vi "HDF5_Init_ADAM_Refs.vi"(5 "HDF5 file ref":T2 format="%.0x", 9 "File Exists?":bool, 11 "error in":errorcluster) -> (4 "Health_Refs":T1 {"Group_ref" format="%.0x"; "ADAM_CoPol_dset" format="%.0x"; "ADAM_XPol_dset" format="%.0x"; "ADAM_Noise_dset" format="%.0x"; "ADAM_CalBox_dset" format="%.0x"; "TimeStamp" format="%.0x"}, 15 "error out":errorcluster)   [LabVIEW 2018]
doc: "Set up the HDF5 data structure and initialize the references for the Noise1, Noise2, Noise3, and Noise4 Datasets (tables).\n\nData structure:\nNoise1 (Dataset) - 1024 element Double array (waveform) \nNoise2 (Dataset) - 1024 element Double array (waveform) \nNoise3 (Dataset) - 1024 element Double array (waveform) \nNoise4 (Dataset) - 1024 element Double array (waveform)"
uses:
  <vilib>/addons/h5labview2/base/hid_t.ctl
  HDF5_ADAM_Refs.ctl
  HDF5_ADAM_Data.ctl
  lib_path_mod_20200519.vi
  <vilib>/addons/h5labview2/base/H5Equery.vi
  <vilib>/addons/h5labview2/attrib/H5Awrite.llb/H5Awrite.xnode
  <vilib>/addons/h5labview2/group/H5G.lvlib
  <vilib>/addons/h5labview2/dataset/H5D.lvlib
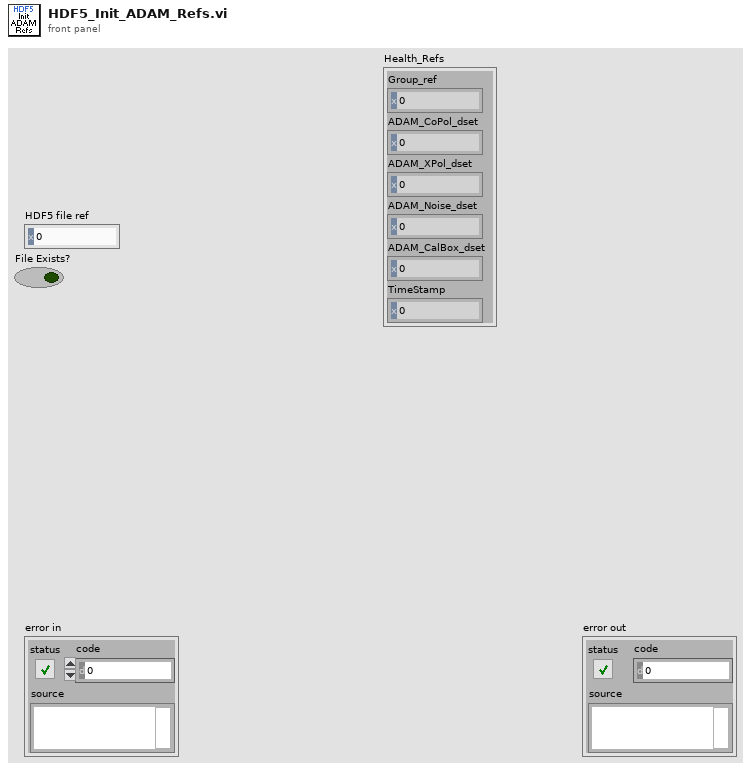
[diagram p1: front panel]
types:
  T1 = typedef "HDF5_ADAM_Refs.ctl" = cluster{"Group_ref":T2, "ADAM_CoPol_dset":T2, "ADAM_XPol_dset":T2, "ADAM_Noise_dset":T2, "ADAM_CalBox_dset":T2, "TimeStamp":T2}
  T2 = typedef "hid_t.ctl" = i32
  T3 = typedef "HDF5_ADAM_Data.ctl" = cluster{"Timestamp":dbl, "Time string":string, "Fault 1":bool, "Fault 2":bool, "Fault 3":bool, "Fault 4":bool, "Fault 5":bool, "Fault 6":bool, "Value 1":dbl, "Value 2":dbl, "Value 3":dbl, "Value 4":dbl, "Value 5":dbl, "Value 6":dbl}
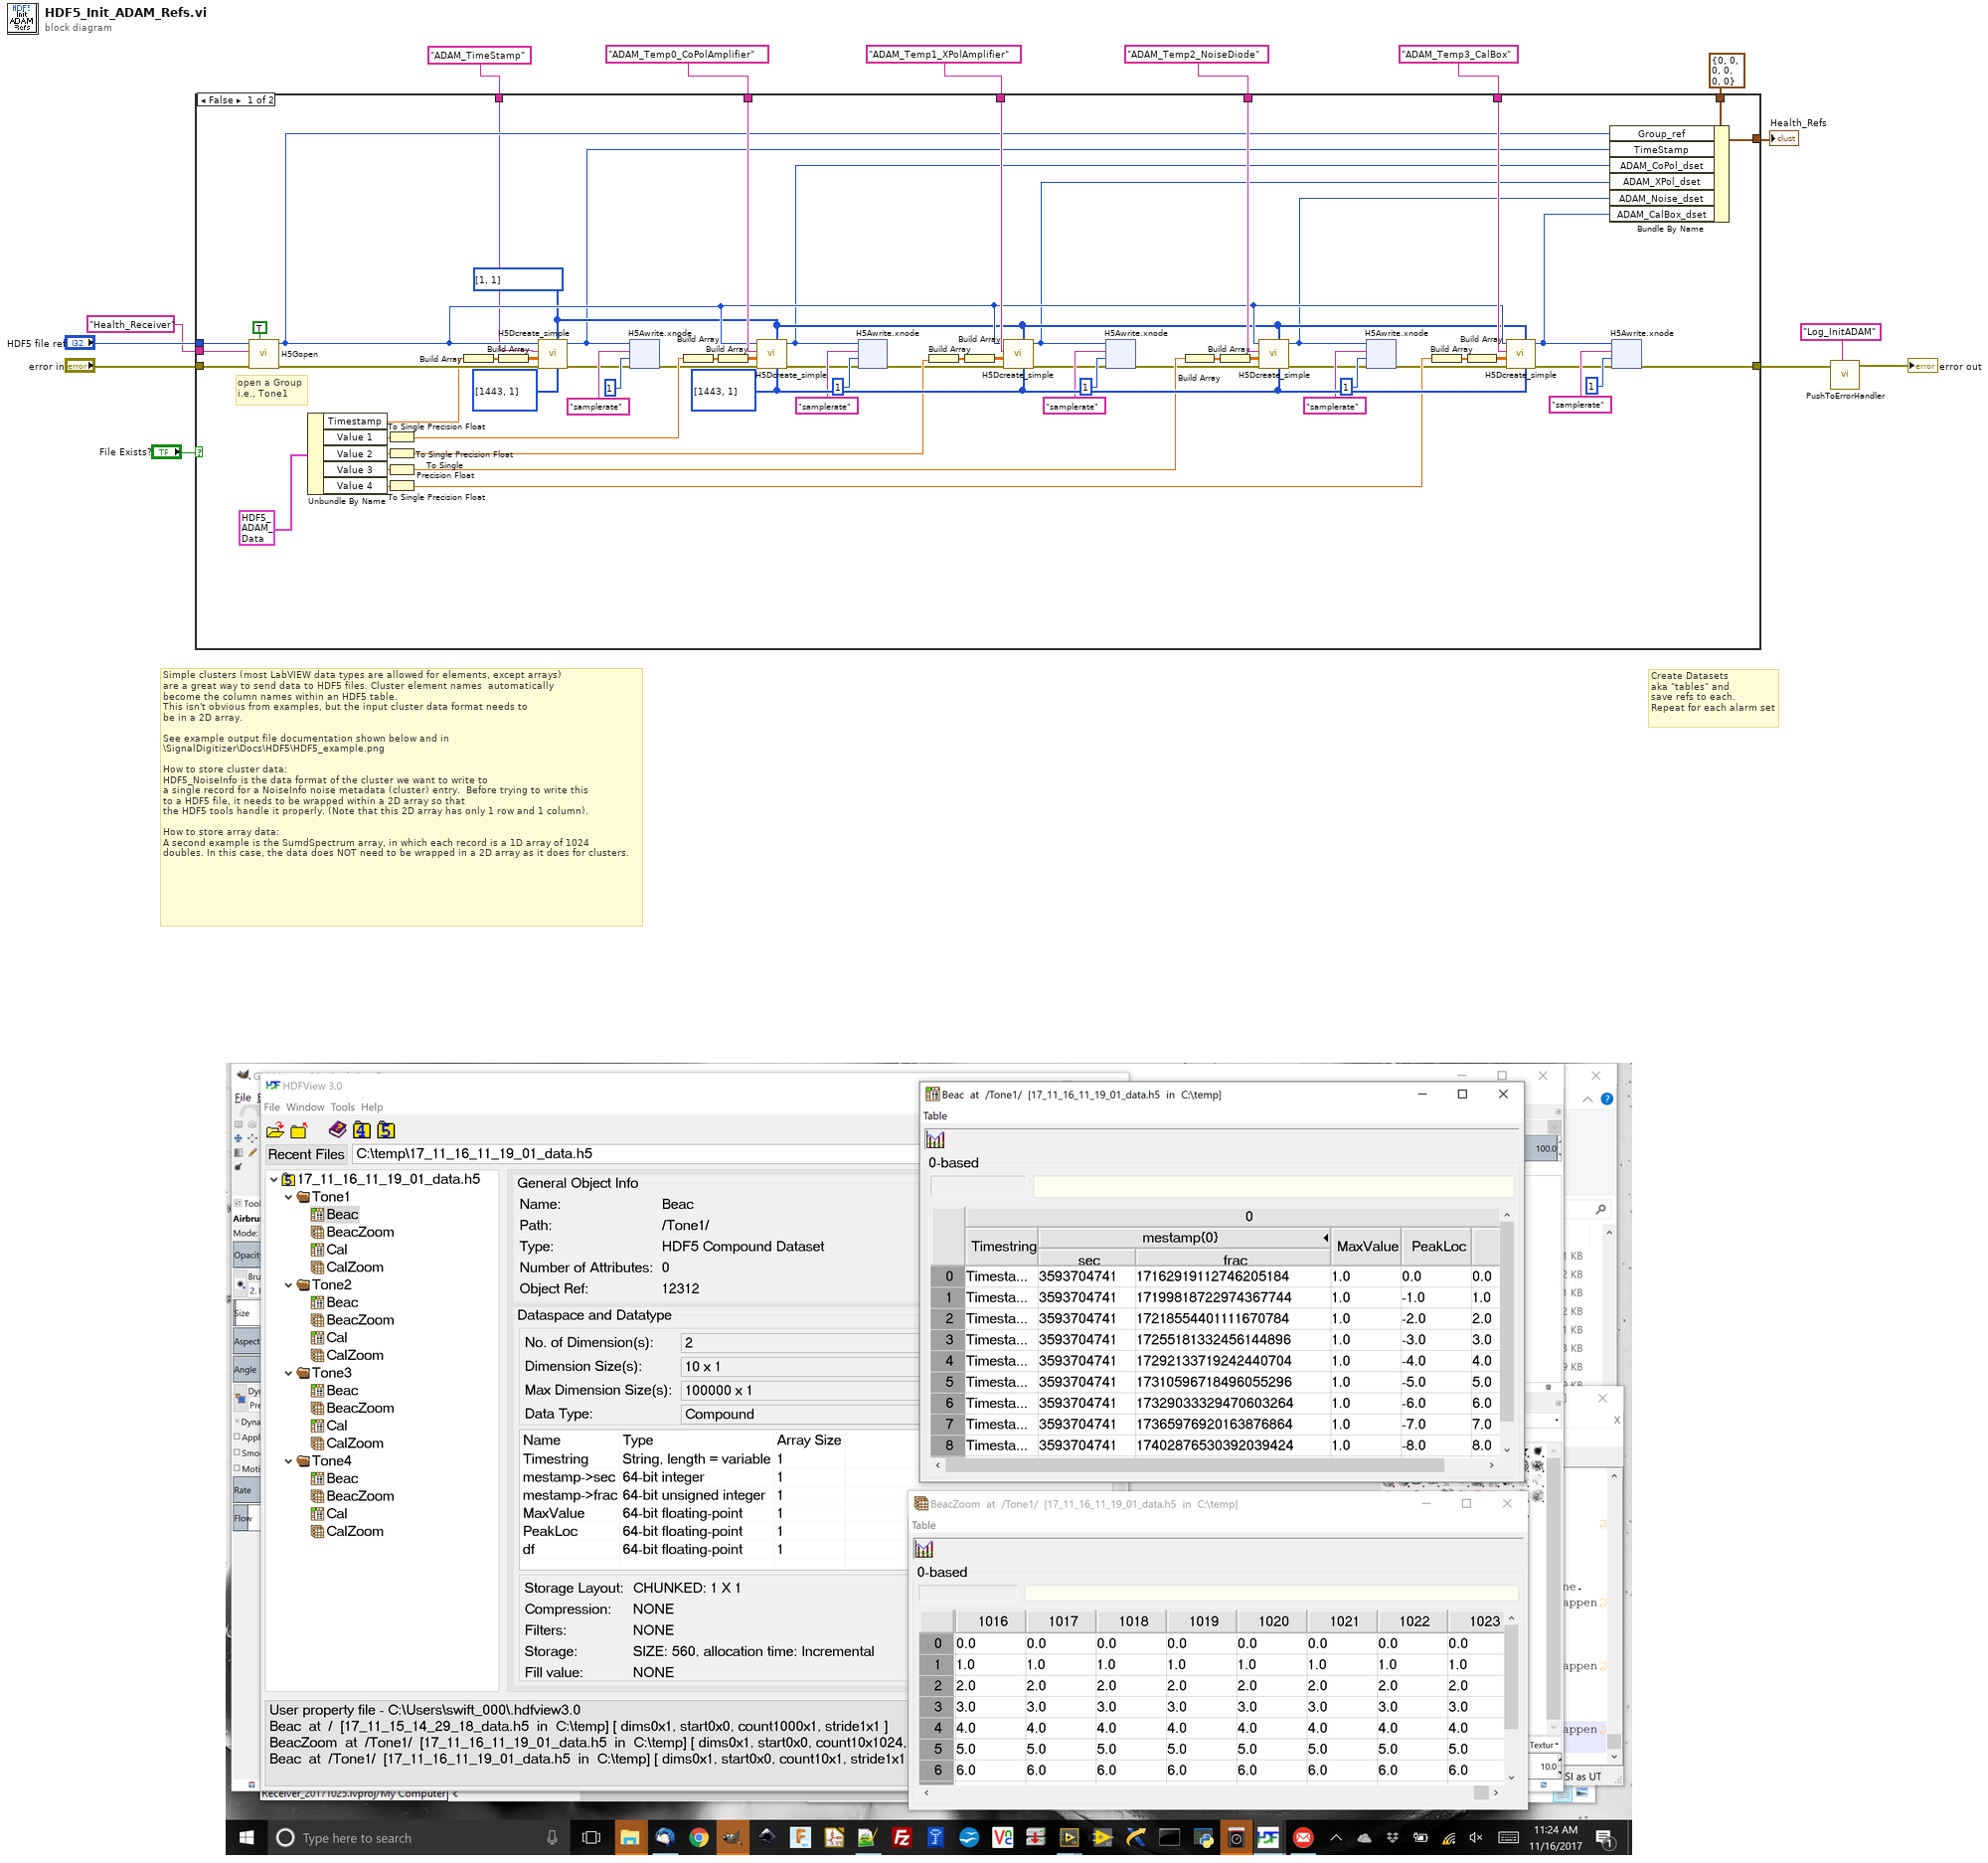
[diagram p0: block diagram]
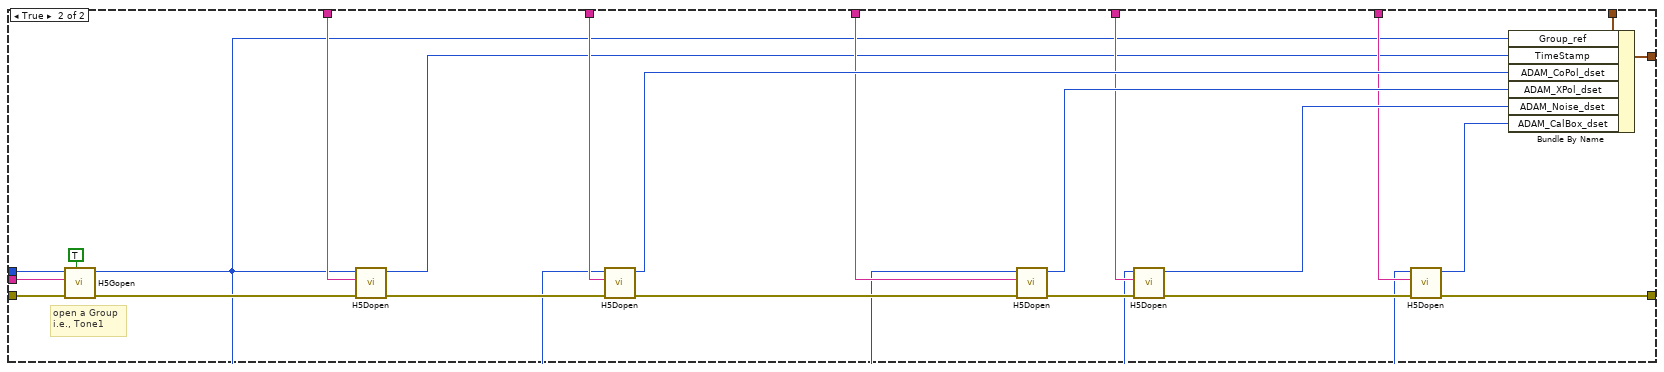
[diagram p2: hidden frame]
diagram:
  # "Create Datasets\naka \"tables\" and\nsave refs to each.\nRepeat for each alarm set"
  # "Simple clusters (most LabVIEW data types are allowed for elements, except arrays) \nare a great way to send data to HDF5 files. Cluster element names  automatically\nbecome the column names within an HDF5 table.\nThis isn't obvious from examples, but the input cluster data format needs to \nbe in a 2D array.\n\nSee example output file documentation shown below and in\n\\SignalDigitizer\\Docs\\HDF5\\HDF5_example.png\n\nHow to store cluster data:\nHDF5_NoiseInfo is the data format of the cluster we want to write to \na single record for a NoiseInfo noise metadata (cluster) entry.  Before trying to write this \nto a HDF5 file, it needs to be wrapped within a 2D array so that \nthe HDF5 tools handle it properly. (Note that this 2D array has only 1 row and 1 column).\n\nHow to store array data:\nA second example is the SumdSpectrum array, in which each record is a 1D array of 1024 \ndoubles. In this case, the data does NOT need to be wrapped in a 2D array as it does for clusters."
  n1 = case shown="False" "File Exists?" {
    tunnel: "error in" -> [w75 w193]
    tunnel: "HDF5 file ref" -> [w74 w192]
    tunnel: T1 {"Group_ref"=0, "ADAM_CoPol_dset"=0, "ADAM_XPol_dset"=0, "ADAM_Noise_dset"=0, "ADAM_CalBox_dset"=0, "TimeStamp"=0} ("Health_Refs") -> [w70 w190]
    tunnel: "ADAM_Temp0_CoPolAmplifier" ("string") -> [w69 w188]
    tunnel: "Health_Receiver" ("name") -> [w68 w187]
    tunnel: [w67 w186] -> w4
    tunnel: [w15 w176] -> w3
    tunnel: "ADAM_Temp1_XPolAmplifier" ("string") -> [w59 w179]
    tunnel: "ADAM_Temp2_NoiseDiode" ("string") -> [w58 w178]
    tunnel: "ADAM_Temp3_CalBox" ("string") -> [w57 w177]
    tunnel: "ADAM_TimeStamp" ("name") -> [w42 w173]
    frame False {
      w43 = i32[] [1, 1] ("size(s)")
      w56 = u64[] [1443, 1] ("max size")
      # "open a Group\ni.e., Tone1"
      n2 = call <vilib>:"H5Gopen.vi"("create? (F)"=TRUE, "error in (no error)"=w75, "name"=w68, "ref in"=w74) -> ("error out"=w45:errorcluster, "group out"=w44:T2)  [unwired: 6 in]
      n3 = Unbundle By Name(T3 {"Timestamp"=0.0, "Time string"="", "Fault 1"=FALSE, "Fault 2"=FALSE, "Fault 3"=FALSE, "Fault 4"=FALSE, "Fault 5"=FALSE, "Fault 6"=FALSE, "Value 1"=0.0, "Value 2"=0.0, "Value 3"=0.0, "Value 4"=0.0, "Value 5"=0.0, "Value 6"=0.0}) -> ("Timestamp"=w41:dbl, "Value 1"=w66:dbl, "Value 2"=w51:dbl, "Value 3"=w50:dbl, "Value 4"=w49:dbl)
      n4 = To Single Precision Float(number=w66) -> (single precision float=w55:sgl)
      n5 = To Single Precision Float(number=w51) -> (single precision float=w54:sgl)
      n6 = To Single Precision Float(number=w50) -> (single precision float=w53:sgl)
      n7 = To Single Precision Float(number=w49) -> (single precision float=w52:sgl)
      n8 = Build Array(w41) -> (w46:dbl[])
      n9 = Build Array(w46) -> (w47:dbl[][])
      n10 = call <vilib>:"H5Dcreate_simple.vi"("max size"=u64[] [1443, 1], "chunk size"=w43, "error in (no error)"=w45, "type in"=w47, "name"=w42, "ref in"=w44) -> ("error out"=w37:errorcluster, "dset out"=w36:T2)  [unwired: 4 in]
      n11 = xnode "H5Awrite.xnode"("error in (no error)"=w37, "data"=u32 1, "attrib name"="samplerate", "ref in"=w36) -> ("error out"=w35:errorcluster)  [unwired: 3 in, 2 out]
      n12 = Build Array(w55) -> (w73:sgl[])
      n13 = Build Array(w73) -> (w72:sgl[][])
      n14 = call <vilib>:"H5Dcreate_simple.vi"("max size"=w56, "chunk size"=w43, "error in (no error)"=w35, "type in"=w72, "name"=w69, "ref in"=w44) -> ("error out"=w32:errorcluster, "dset out"=w31:T2)  [unwired: 4 in]
      n15 = xnode "H5Awrite.xnode"("error in (no error)"=w32, "data"=u32 1, "attrib name"="samplerate", "ref in"=w31) -> ("error out"=w30:errorcluster)  [unwired: 3 in, 2 out]
      n16 = Build Array(w54) -> (w64:sgl[])
      n17 = Build Array(w64) -> (w65:sgl[][])
      n18 = call <vilib>:"H5Dcreate_simple.vi"("max size"=w56, "chunk size"=w43, "error in (no error)"=w30, "type in"=w65, "name"=w59, "ref in"=w44) -> ("error out"=w27:errorcluster, "dset out"=w26:T2)  [unwired: 4 in]
      n19 = xnode "H5Awrite.xnode"("error in (no error)"=w27, "data"=u32 1, "attrib name"="samplerate", "ref in"=w26) -> ("error out"=w25:errorcluster)  [unwired: 3 in, 2 out]
      n20 = Build Array(w53) -> (w63:sgl[])
      n21 = Build Array(w63) -> (w62:sgl[][])
      n22 = call <vilib>:"H5Dcreate_simple.vi"("max size"=w56, "chunk size"=w43, "error in (no error)"=w25, "type in"=w62, "name"=w58, "ref in"=w44) -> ("error out"=w22:errorcluster, "dset out"=w21:T2)  [unwired: 4 in]
      n23 = xnode "H5Awrite.xnode"("error in (no error)"=w22, "data"=u32 1, "attrib name"="samplerate", "ref in"=w21) -> ("error out"=w20:errorcluster)  [unwired: 3 in, 2 out]
      n24 = Build Array(w52) -> (w60:sgl[])
      n25 = Build Array(w60) -> (w61:sgl[][])
      n26 = call <vilib>:"H5Dcreate_simple.vi"("max size"=w56, "chunk size"=w43, "error in (no error)"=w20, "type in"=w61, "name"=w57, "ref in"=w44) -> ("error out"=w17:errorcluster, "dset out"=w16:T2)  [unwired: 4 in]
      n27 = Bundle By Name(cluster=w70, "Group_ref"=w44, "TimeStamp"=w36, "ADAM_CoPol_dset"=w31, "ADAM_XPol_dset"=w26, "ADAM_Noise_dset"=w21, "ADAM_CalBox_dset"=w16) -> (w67:T1)
      n28 = xnode "H5Awrite.xnode"("error in (no error)"=w17, "data"=u32 1, "attrib name"="samplerate", "ref in"=w16) -> ("error out"=w15:errorcluster)  [unwired: 3 in, 2 out]
    }
    frame True {
      # "open a Group\ni.e., Tone1"
      n29 = call <vilib>:"H5Gopen.vi"("create? (F)"=TRUE, "error in (no error)"=w193, "name"=w187, "ref in"=w192) -> ("error out"=w175:errorcluster, "group out"=w172:T2)  [unwired: 6 in]
      n30 = call <vilib>:"H5Dopen.vi"("error in (no error)"=w175, "name"=w173, "loc in"=w172) -> ("error out"=w174:errorcluster, "dset out"=w171:T2)  [unwired: 7 in]
      n31 = call <vilib>:"H5Dopen.vi"("error in (no error)"=w174, "name"=w188, "loc in"=w172) -> ("error out"=w185:errorcluster, "dset out"=w189:T2)  [unwired: 7 in]
      n32 = call <vilib>:"H5Dopen.vi"("error in (no error)"=w185, "name"=w179, "loc in"=w172) -> ("error out"=w184:errorcluster, "dset out"=w180:T2)  [unwired: 7 in]
      n33 = call <vilib>:"H5Dopen.vi"("error in (no error)"=w184, "name"=w178, "loc in"=w172) -> ("error out"=w183:errorcluster, "dset out"=w181:T2)  [unwired: 7 in]
      n34 = call <vilib>:"H5Dopen.vi"("error in (no error)"=w183, "name"=w177, "loc in"=w172) -> ("error out"=w176:errorcluster, "dset out"=w182:T2)  [unwired: 7 in]
      n35 = Bundle By Name(cluster=w190, "Group_ref"=w172, "TimeStamp"=w171, "ADAM_CoPol_dset"=w189, "ADAM_XPol_dset"=w180, "ADAM_Noise_dset"=w181, "ADAM_CalBox_dset"=w182) -> (w186:T1)
    }
  }
  "Health_Refs" <- w4
  n36 = call "PushToErrorHandler.vi"("ErrorIn"=w3, "ErrorLocation"="Log_InitADAM") -> ("ErrorOut"=→"error out":errorcluster)  [unwired: 5 in]
